vi "SetDefaultColumnHeaders.vi"(8 "error in (no error)":errorcluster, 11 "ResultTree in":refnum<class "ResultTree.lvclass">) -> (0 "error out":errorcluster, 3 "ResultTree out":refnum<class "ResultTree.lvclass">)   [LabVIEW 2017, in "ResultTree.lvclass"]
doc: "Sets the default column headers."
uses:
  ResultTree.lvclass
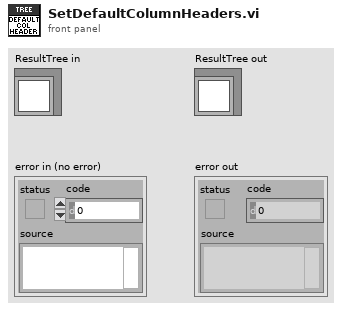
[diagram p1: front panel]
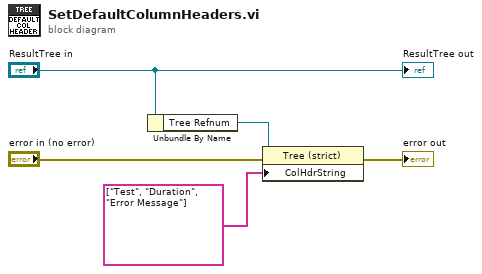
[diagram p0: block diagram]
diagram:
  n1 = Unbundle By Name("ResultTree in") -> ("Tree Refnum"=w2:refnum<vi>)
  n2 = property class="Tree (strict)"(reference=w2, error in="error in (no error)", "ColHdrString"=string[] ["Test", "Duration", "Error Message"] ("Column Header Strings[]")) -> (error out=→"error out":errorcluster)  [unwired: 1 out]
  "ResultTree out" <- "ResultTree in"
